vi "Create-Destroy.vi"(8 "Error In":errorcluster) -> (0 "Error Out":errorcluster)   [LabVIEW 2018, in "Tests.lvlib" / "SFTP Attributes.lvlib"]
uses:
  SFTP Attributes.lvlib
  src/Toolkit/SFTP Attributes/Support/Create from SSH.vi
  src/Toolkit/SFTP Attributes/Support/Destroy to SSH.vi
  <vilib>/addons/_JKI Toolkits/Caraya/classes/Test/Test.lvclass
  src/Toolkit/SSH/SSH.lvclass
  <vilib>/addons/_JKI Toolkits/Caraya/classes/Assert/Assert.lvclass
  src/Toolkit/SFTP Attributes/SFTP Attributes.lvclass
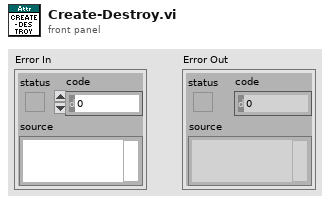
[diagram p1: front panel]
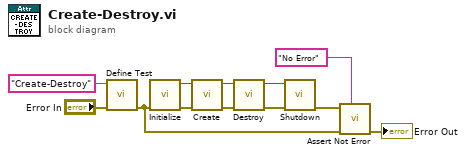
[diagram p0: block diagram]
diagram:
  n1 = call <vilib>:"Define Test.vi"("error in (no error)"="Error In", "Label (VI Title)"="Create-Destroy") -> ("error out"=w8:errorcluster)  [unwired: 9 in]
  n2 = call "Initialize.vi"("Error In"=w8) -> ("Error Out"=w6:errorcluster, "SSH"=w5:refnum<class "SSH.lvclass">)  [unwired: 9 in]
  n3 = call-poly "Create.vi"("Error In"=w6, "SSH"=w5) -> ("Error Out"=w3:errorcluster, "SFTP Attributes"=w4:refnum<class "SFTP Attributes.lvclass">)  [unwired: 8 in]
  n4 = call-poly "Destroy.vi"("Error In"=w3, "SFTP Attributes"=w4) -> ("Error Out"=w1:errorcluster, "SSH"=w2:refnum<class "SSH.lvclass">)  [unwired: 8 in]
  n5 = call "Shutdown.vi"("Error In"=w1, "SSH"=w2) -> ("Error Out"=w10:errorcluster)  [unwired: 9 in]
  n6 = call <vilib>:"Assert Not Error.vi"("Label"="No Error", "error in (no error)"=w8, "Not Error?"=w10) -> ("error out"=→"Error Out":errorcluster)  [unwired: 8 in]
